vi "Write reinitializeIsTrue.vi"(10 "reinitializeIsTrue":bool, 11 "SystemController in":refnum<class "SystemController.lvclass">) -> (3 "SystemController out":refnum<class "SystemController.lvclass">)   [LabVIEW 2015]
uses:
  SystemController.lvclass
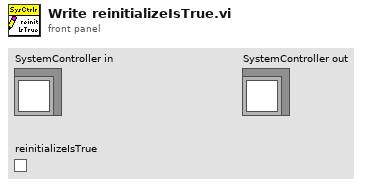
[diagram p1: front panel]
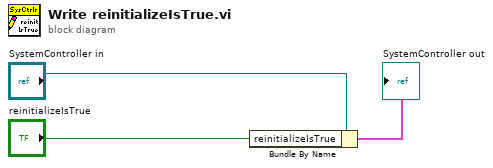
[diagram p0: block diagram]
diagram:
  n1 = Bundle By Name(cluster="SystemController in", "reinitializeIsTrue"="reinitializeIsTrue") -> (→"SystemController out":cluster{})
